vi "Led Power Sliders.vi"() -> ()   [LabVIEW 2014]
uses:
  <vilib>/myRIO/Instrument Drivers/Onboard IO/PWM/typedefs/PWM Reference.ctl
  <vilib>/myRIO/Common/Instrument Driver Framework/Utilities/typedefs/myRIO Generic Hardware Reference.ctl
  <vilib>/myRIO/Common/Instrument Driver Framework/Utilities/typedefs/Hardware Version Enum.ctl
  <vilib>/myRIO/Common/Instrument Driver Framework/Utilities/typedefs/myRIO v1.0 Reference.ctl
  <vilib>/myRIO/Common/Instrument Driver Framework/Utilities/typedefs/Generic FPGA Reference.ctl
  <vilib>/myRIO/Common/Instrument Driver Framework/myRIO v1.0/PWM/typedefs/PWM Channels Enum.ctl
  <vilib>/myRIO/Instrument Drivers/Onboard IO/PWM/typedefs/PWM Configuration.ctl
  <vilib>/userdefined/High Color/nirio_resource_hc.ctl
  <vilib>/myRIO/Instrument Drivers/Onboard IO/I2C/typedefs/I2C User Configuration.ctl
  <vilib>/myRIO/Instrument Drivers/Onboard IO/I2C/typedefs/I2C Transfer Rate.ctl
  <vilib>/myRIO/Instrument Drivers/Onboard IO/I2C/typedefs/I2C Reference.ctl
  <vilib>/myRIO/Common/Instrument Driver Framework/myRIO v1.0/I2C/typedefs/I2C Channels Enum.ctl
  <vilib>/myRIO/Instrument Drivers/Onboard IO/I2C/typedefs/I2C Configuration.ctl
  <vilib>/myRIO/Common/Instrument Driver Framework/Utilities/vis/Is FPGA Ref Available.vi
  <vilib>/myRIO/Common/Instrument Driver Framework/myRIO v1.0/I2C/vis/myRIO v1.1 Open I2C.vi
  <vilib>/myRIO/Instrument Drivers/Onboard IO/I2C/vis/Configure.vi
  <vilib>/myRIO/Instrument Drivers/Onboard IO/I2C/vis/Write.vi
  <vilib>/myRIO/Common/Instrument Driver Framework/myRIO v1.0/PWM/vis/myRIO v1.1 Open PWM.vi
  <vilib>/myRIO/Instrument Drivers/Onboard IO/PWM/vis/Set Duty Cycle and Frequency.vi
  <vilib>/myRIO/Instrument Drivers/Onboard IO/I2C/vis/Write Read.vi
  <vilib>/myRIO/Common/Instrument Driver Framework/Utilities/vis/Validate Channels.vi
  <vilib>/myRIO/Common/Instrument Driver Framework/myRIO v1.0/I2C/vis/myRIO v1.0 Reserve I2C.vi
  <vilib>/myRIO/Common/Instrument Driver Framework/myRIO v1.0/PWM/vis/myRIO v1.0 Reserve PWM.vi
  <vilib>/myRIO/Common/Instrument Driver Framework/myRIO v1.0/I2C/vis/myRIO v1.0 Build MUX Configuration I2C.vi
  <vilib>/myRIO/Common/Instrument Driver Framework/myRIO v1.0/Resource Manager/vis/myRIO v1.0 Reserve Channel List.vi
  <vilib>/myRIO/Common/Instrument Driver Framework/myRIO v1.0/PWM/vis/myRIO v1.0 Build MUX Configuration PWM.vi
  <vilib>/myRIO/Common/Instrument Driver Framework/myRIO v1.0/Resource Manager/vis/myRIO v1.0 Create Configuration List.vi
  <vilib>/myRIO/Common/Instrument Driver Framework/myRIO v1.0/Resource Manager/vis/myRIO v1.0 Reserve Channel.vi
  <vilib>/myRIO/Common/Instrument Driver Framework/myRIO v1.0/Resource Manager/vis/myRIO v1.0 Unreserve Channel.vi
  <vilib>/myRIO/Common/Instrument Driver Framework/myRIO v1.0/Resource Manager/vis/myRIO v1.0 Build Mutex Name.vi
  <vilib>/Utility/VariantDataType/GetNumericInfo.vi
  <vilib>/Utility/error.llb/Error Cluster From Error Code.vi
  <vilib>/myRIO/Common/Instrument Driver Framework/myRIO v1.0/myRIO v1.1 Open.vi
  <vilib>/myRIO/Common/Instrument Driver Framework/Utilities/vis/IO Manager.vi
  <vilib>/myRIO/Common/Instrument Driver Framework/Utilities/vis/Configuration Manager.vi
  <vilib>/myRIO/Common/Instrument Driver Framework/myRIO v1.0/Resource Manager/vis/myRIO v1.0 Configure IO.vi
  <vilib>/myRIO/Common/Instrument Driver Framework/myRIO v1.0/myRIO v1.0 Close.vi
  <vilib>/myRIO/Common/Instrument Driver Framework/myRIO v1.0/PWM/vis/myRIO v1.0 Write PWM.vi
  <vilib>/myRIO/Common/Instrument Driver Framework/myRIO v1.0/I2C/vis/myRIO v1.0 Configure I2C.vi
  <vilib>/myRIO/Common/Instrument Driver Framework/myRIO v1.0/I2C/vis/myRIO v1.0 Write I2C.vi
  <vilib>/myRIO/Common/Instrument Driver Framework/myRIO v1.0/I2C/vis/myRIO v1.0 Read I2C.vi
  <vilib>/myRIO/Express VI/Onboard IO/PWM/PWM Express VI.xnode
  <vilib>/myRIO/Instrument Drivers/Onboard IO/PWM/vis/myRIO PWM Open.xnode
  <vilib>/myRIO/Express VI/Onboard IO/I2C/I2C Express VI.xnode
  <vilib>/myRIO/Instrument Drivers/Onboard IO/I2C/vis/myRIO I2C Open.xnode
  <vilib>/myRIO/Instrument Drivers/Onboard IO/I2C/I2C.lvlib
  <vilib>/myRIO/Instrument Drivers/Onboard IO/PWM/PWM.lvlib
panel:
  out "number (0 to 1)":dbl
  out "Bytes Read":u8[](array[numeric])
  in  "Light":bool
  out "I2C Error?":errorcluster
  out "Clear Reading":u16
  out "Red Reading":u16
  out "Green Reading":u16
  out "Blue Reading":u16
  in  "Stop Run":bool
  in  "Blue LED\nDuty Cycle":dbl(slide) scale=0.0..0.95
  in  "White LED\nDuty Cycle":dbl(slide) scale=0.0..0.9
  in  "Violet LED\nDuty Cycle":dbl(slide) scale=0.0..1.0
  in  "Green LED\nDuty Cycle":dbl(slide) scale=0.0..0.9
  in  "Amber LED\nDuty Cycle":dbl(slide) scale=0.0..0.65
  in  "Red LED\nDuty Cycle":dbl(slide) scale=0.0..0.6
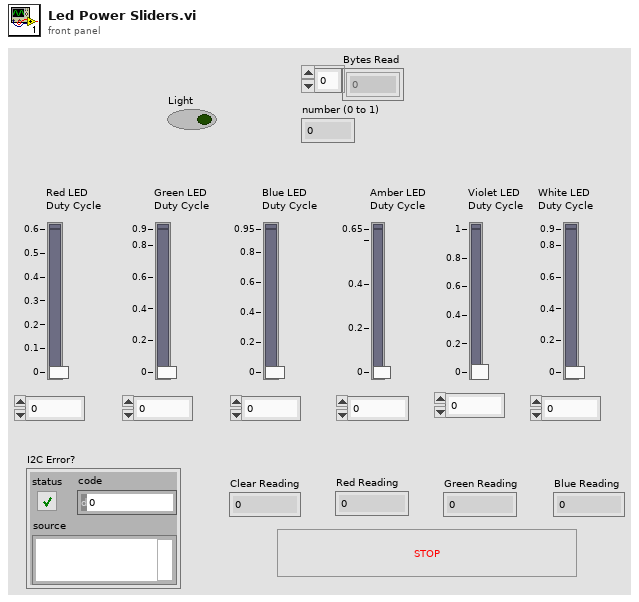
[diagram p1: front panel]
types:
  T1 = typedef "I2C.lvlib/I2C Reference.ctl" = cluster{"myRIO Reference":T2, "I2C Channels Enum":T6, "I2C Configuration":T7}
  T2 = typedef "myRIO Generic Hardware Reference.ctl" = cluster{"myRIO Model":T3, "myRIO Hardware Reference":T4}
  T3 = typedef "Hardware Version Enum.ctl" = enum16{"Unknown", "myRIO-1900", "myRIO-1950"}
  T4 = typedef "myRIO v1.0 Reference.ctl" = cluster{"Generic FPGA Reference":T5, "Allow multiple opens":bool}
  T5 = typedef "Generic FPGA Reference.ctl" = refnum<k20>
  T6 = typedef "I2C Channels Enum.ctl" = enum16{"Not Connected", "A/I2C", "B/I2C"}
  T7 = typedef "I2C.lvlib/I2C Configuration.ctl" = cluster{"I2C Transfer Rate":T8}
  T8 = typedef "I2C.lvlib/I2C Transfer Rate.ctl" = enum16{"Standard mode (100 kbps)", "Fast mode (400 kbps)"}
  T9 = typedef "I2C.lvlib/I2C User Configuration.ctl" = cluster{"I2C Transfer Rate":T8}
  T10 = typedef "nirio_resource_hc.ctl" = tag
  T11 = typedef "PWM.lvlib/PWM Reference.ctl" = cluster{"myRIO Reference":T2, "PWM Channels Enum":T12, "PWM Configuration":T13}
  T12 = typedef "PWM Channels Enum.ctl" = enum16{"Not Connected", "C/PWM0", "C/PWM1", "A/PWM0", "A/PWM1", "A/PWM2", "B/PWM0", "B/PWM1", "B/PWM2"}
  T13 = typedef "PWM.lvlib/PWM Configuration.ctl" = cluster{"Frequency":dbl, "Duty Cycle":dbl}
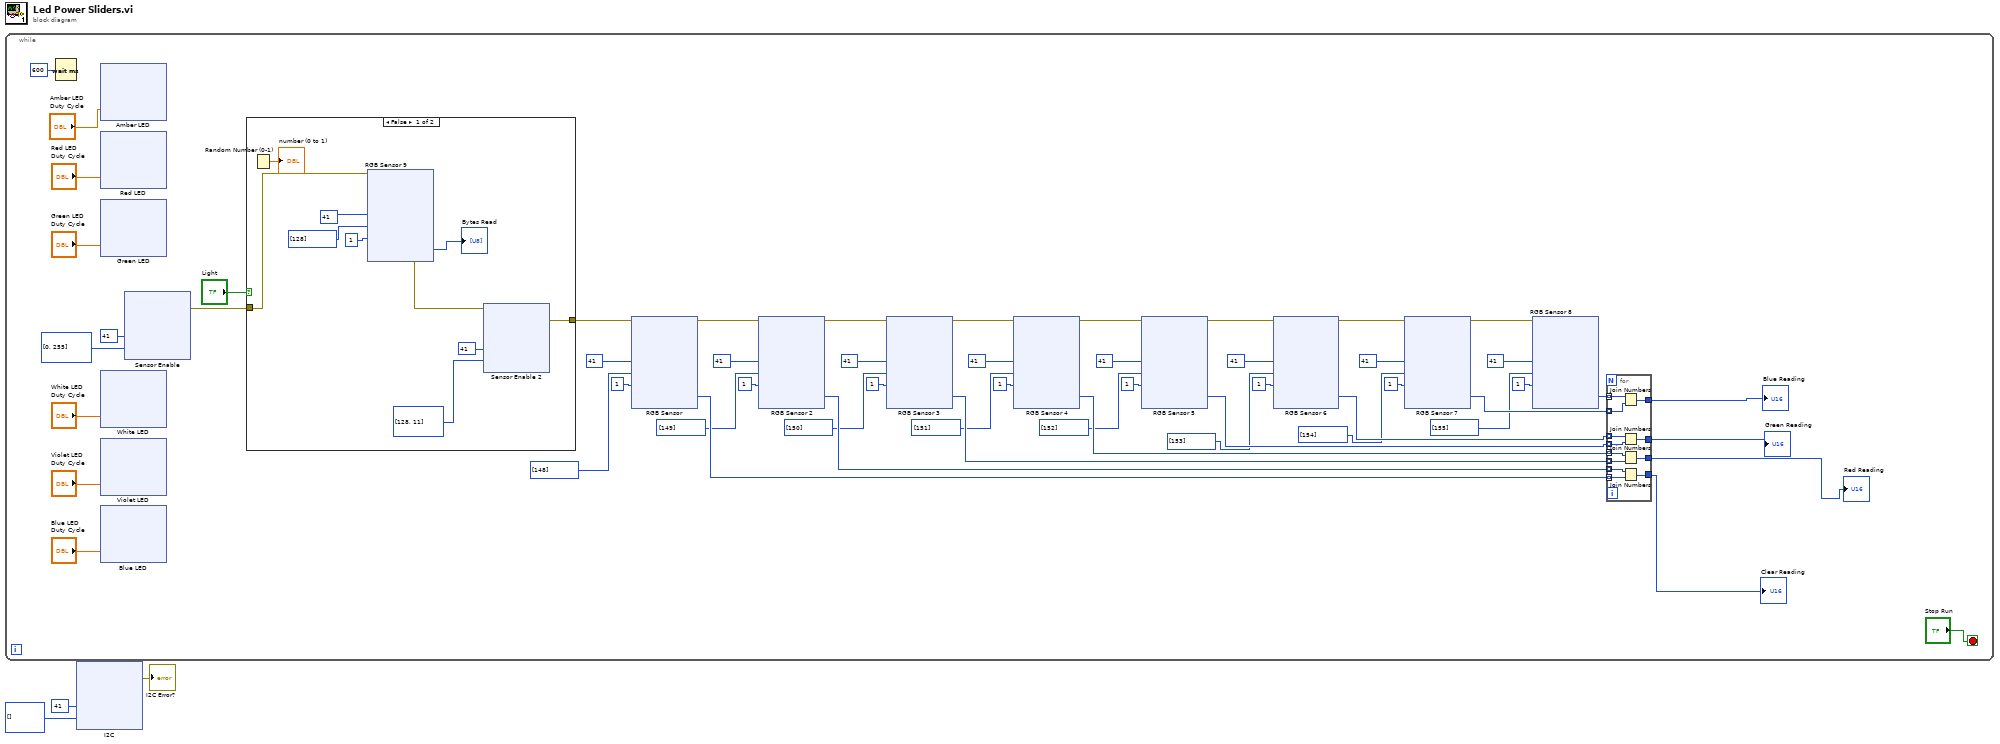
[diagram p0: block diagram]
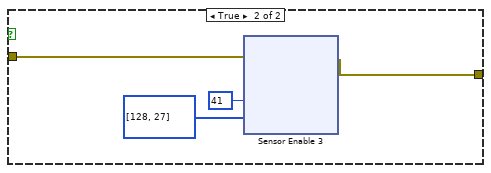
[diagram p2: hidden frame]
diagram:
  n1 = while {
    stop <- "Stop Run" stop-if-true
    n2 = Wait (ms)(milliseconds to wait=u32 600) -> ()  [unwired: 1 out]
    n3 = xnode "Amber LED"("Duty Cycle"="Amber LED\nDuty Cycle") -> ()  [unwired: 1 in, 1 out]
    n4 = xnode "Red LED"("Duty Cycle"="Red LED\nDuty Cycle") -> ()  [unwired: 1 in, 1 out]
    n5 = xnode "Green LED"("Duty Cycle"="Green LED\nDuty Cycle") -> ()  [unwired: 1 in, 1 out]
    n6 = xnode "White LED"("Duty Cycle"="White LED\nDuty Cycle") -> ()  [unwired: 1 in, 1 out]
    n7 = xnode "Violet LED"("Duty Cycle"="Violet LED\nDuty Cycle") -> ()  [unwired: 1 in, 1 out]
    n8 = xnode "Blue LED"("Duty Cycle"="Blue LED\nDuty Cycle") -> ()  [unwired: 1 in, 1 out]
    n9 = xnode "Sensor Enable"("Slave Address (7-bit)"=u8 41, "Bytes to Write"=u8[] [0, 255]) -> ("error out"=w10:errorcluster)  [unwired: 1 in]
    n10 = case shown="False" "Light" {
      tunnel: w10 -> [w61 w149]
      tunnel: [w60 w148] -> w9
      frame False {
        n11 = Random Number (0-1)() -> (number: 0 to 1=→"number (0 to 1)":dbl)
        n12 = xnode "RGB Sensor 9"("Slave Address (7-bit)"=u8 41, "Bytes to Write"=u8[] [128], "Byte Count"=u32 1, "error in (no error)"=w61) -> ("Bytes Read"=→"Bytes Read":u8[], "error out"=w62:errorcluster)
        n13 = xnode "Sensor Enable 2"("Slave Address (7-bit)"=u8 41, "Bytes to Write"=u8[] [128, 11], "error in (no error)"=w62) -> ("error out"=w60:errorcluster)
      }
      frame True {
        n14 = xnode "Sensor Enable 3"("Slave Address (7-bit)"=u8 41, "Bytes to Write"=u8[] [128, 27], "error in (no error)"=w149) -> ("error out"=w148:errorcluster)
      }
    }
    n15 = xnode "RGB Sensor"("Slave Address (7-bit)"=u8 41, "Bytes to Write"=u8[] [148], "Byte Count"=u32 1, "error in (no error)"=w9) -> ("Bytes Read"=w48:u8[], "error out"=w41:errorcluster)
    n16 = xnode "RGB Sensor 2"("Slave Address (7-bit)"=u8 41, "Bytes to Write"=u8[] [149], "Byte Count"=u32 1, "error in (no error)"=w41) -> ("Bytes Read"=w49:u8[], "error out"=w42:errorcluster)
    n17 = xnode "RGB Sensor 3"("Slave Address (7-bit)"=u8 41, "Bytes to Write"=u8[] [150], "Byte Count"=u32 1, "error in (no error)"=w42) -> ("Bytes Read"=w50:u8[], "error out"=w43:errorcluster)
    n18 = xnode "RGB Sensor 4"("Slave Address (7-bit)"=u8 41, "Bytes to Write"=u8[] [151], "Byte Count"=u32 1, "error in (no error)"=w43) -> ("Bytes Read"=w51:u8[], "error out"=w44:errorcluster)
    n19 = xnode "RGB Sensor 5"("Slave Address (7-bit)"=u8 41, "Bytes to Write"=u8[] [152], "Byte Count"=u32 1, "error in (no error)"=w44) -> ("Bytes Read"=w52:u8[], "error out"=w45:errorcluster)
    n20 = xnode "RGB Sensor 6"("Slave Address (7-bit)"=u8 41, "Bytes to Write"=u8[] [153], "Byte Count"=u32 1, "error in (no error)"=w45) -> ("Bytes Read"=w53:u8[], "error out"=w46:errorcluster)
    n21 = xnode "RGB Sensor 7"("Slave Address (7-bit)"=u8 41, "Bytes to Write"=u8[] [154], "Byte Count"=u32 1, "error in (no error)"=w46) -> ("Bytes Read"=w54:u8[], "error out"=w47:errorcluster)
    n22 = xnode "RGB Sensor 8"("Slave Address (7-bit)"=u8 41, "Bytes to Write"=u8[] [155], "Byte Count"=u32 1, "error in (no error)"=w47) -> ("Bytes Read"=w55:u8[])  [unwired: 1 out]
    n23 = for {
      tunnel: [w479] -> w7
      tunnel: w48 -> [w478] mode=indexing
      tunnel: w49 -> [w477] mode=indexing
      tunnel: w50 -> [w476] mode=indexing
      tunnel: w51 -> [w475] mode=indexing
      tunnel: w52 -> [w474] mode=indexing
      tunnel: w53 -> [w473] mode=indexing
      tunnel: w54 -> [w472] mode=indexing
      tunnel: w55 -> [w471] mode=indexing
      tunnel: [w470] -> w6
      tunnel: [w469] -> w5
      tunnel: [w468] -> w4
      n24 = Join Numbers(hi=w471, lo=w472) -> ((hi.lo)=w468:u16)
      n25 = Join Numbers(hi=w473, lo=w474) -> ((hi.lo)=w469:u16)
      n26 = Join Numbers(hi=w475, lo=w476) -> ((hi.lo)=w470:u16)
      n27 = Join Numbers(hi=w477, lo=w478) -> ((hi.lo)=w479:u16)
    }
    "Clear Reading" <- w7
    "Blue Reading" <- w4
    "Red Reading" <- w6
    "Green Reading" <- w5
  }
  n28 = xnode "I2C"("Slave Address (7-bit)"=u8 41, "Bytes to Write"=u8[] []) -> ("error out"=→"I2C Error?":errorcluster)  [unwired: 1 in]
